vi "PH_Beckhoff.get AE.vi"(0 "Analog Inputs":T1, 1 "index of element":i32) -> (2 "DIM value":dbl, 3 "Quality":bool, 4 "Tag not found":bool)   [LabVIEW 2014, in "PH_Beckhoff.lvlib"]
uses:
  PH_Beckhoff.lvlib
  PH_Beckhoff.Analog Inputs.ctl
  PH_Beckhoff.Scaling Type.ctl
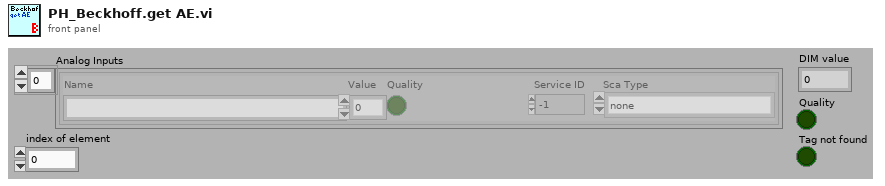
[diagram p1: front panel]
types:
  T1 = typedef "PH_Beckhoff.lvlib/PH_Beckhoff.Analog Inputs.ctl" = cluster{"Name":string, "Value":u32, "Quality":bool, "Service ID":i32, "Sca Type":T2}[]
  T2 = typedef "PH_Beckhoff.lvlib/PH_Beckhoff.Scaling Type.ctl" = enum16{"none", "0 ... 15 Bit -> 0 ... 5", "0 ... 15 Bit -> 0 ... 10", "0 ... 15 Bit -> 0 ... 25", "0 ... 15 Bit -> 4 ... 20", "0 ... 15 Bit -> 0 ... 1", "0 ... 15 Bit -> 0 ... 20000", "0 ... 15 Bit -> 0 ... 24000"}
  T3 = cluster{"Name":string, "Value":u32, "Quality":bool, "Service ID":i32, "Sca Type":T2}
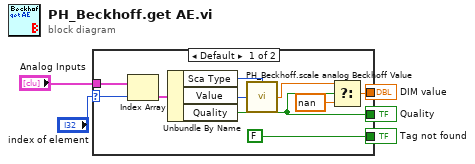
[diagram p0: block diagram]
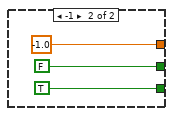
[diagram p2: hidden frame]
diagram:
  n1 = case shown="Default" "index of element" {
    selector: "index of element" -> [w11 _]
    tunnel: [w9 FALSE] -> w3
    tunnel: [w7 -1.0 ("DIM value")] -> w2
    tunnel: "Analog Inputs" -> [w15 _]
    tunnel: [FALSE TRUE] -> w5
    frame Default {
      n2 = Index Array(array=w15, index=w11) -> (element=w14:T3)
      n3 = Unbundle By Name(w14) -> ("Sca Type"=w13:T2, "Value"=w12:u32, "Quality"=w9:bool)
      n4 = call "PH_Beckhoff.scale analog Beckhoff Value.vi"("Beckhoff value"=w12, "Scaling Type"=w13) -> ("DIM value"=w8:dbl)
      n5 = Select(t=w8, s=w9, f=nan) -> (s? t:f=w7:dbl)
    }
    frame -1 {
    }
  }
  "Tag not found" <- w5
  "Quality" <- w3
  "DIM value" <- w2
